vi "GUI_CH1_RXXXX_TCPIP.vi"() -> ()   [LabVIEW 2018]
uses:
  <resource>/objmgr/ni.dex.rc
panel:
  in  "stop 2":bool
  out "error out 3":errorcluster
  out "error out 2":errorcluster
  out "error out":errorcluster
  in  "stop":bool
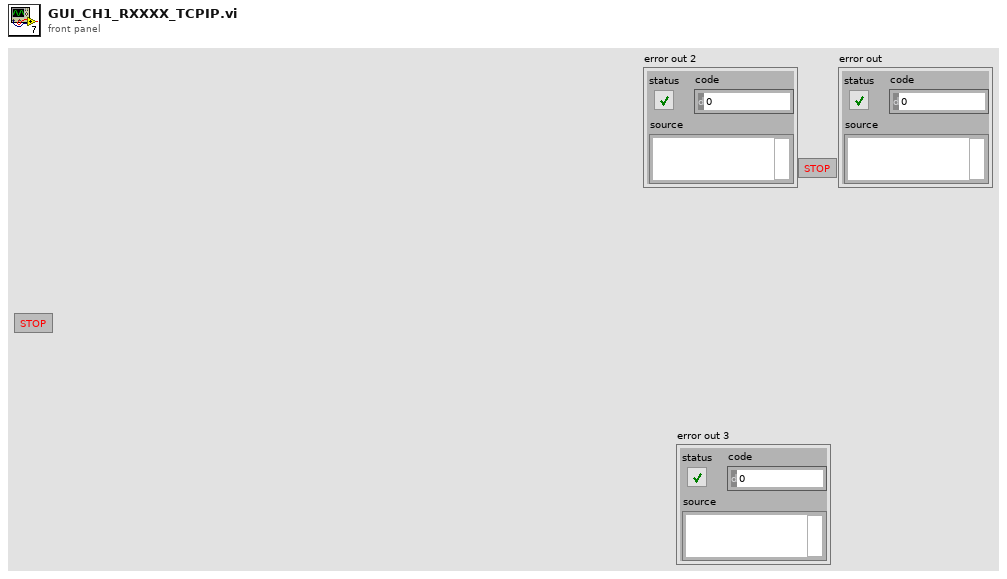
[diagram p1: front panel]
types:
  T1 = enum16{"Standard", "Buffered", "CRLF", "Immediate"}
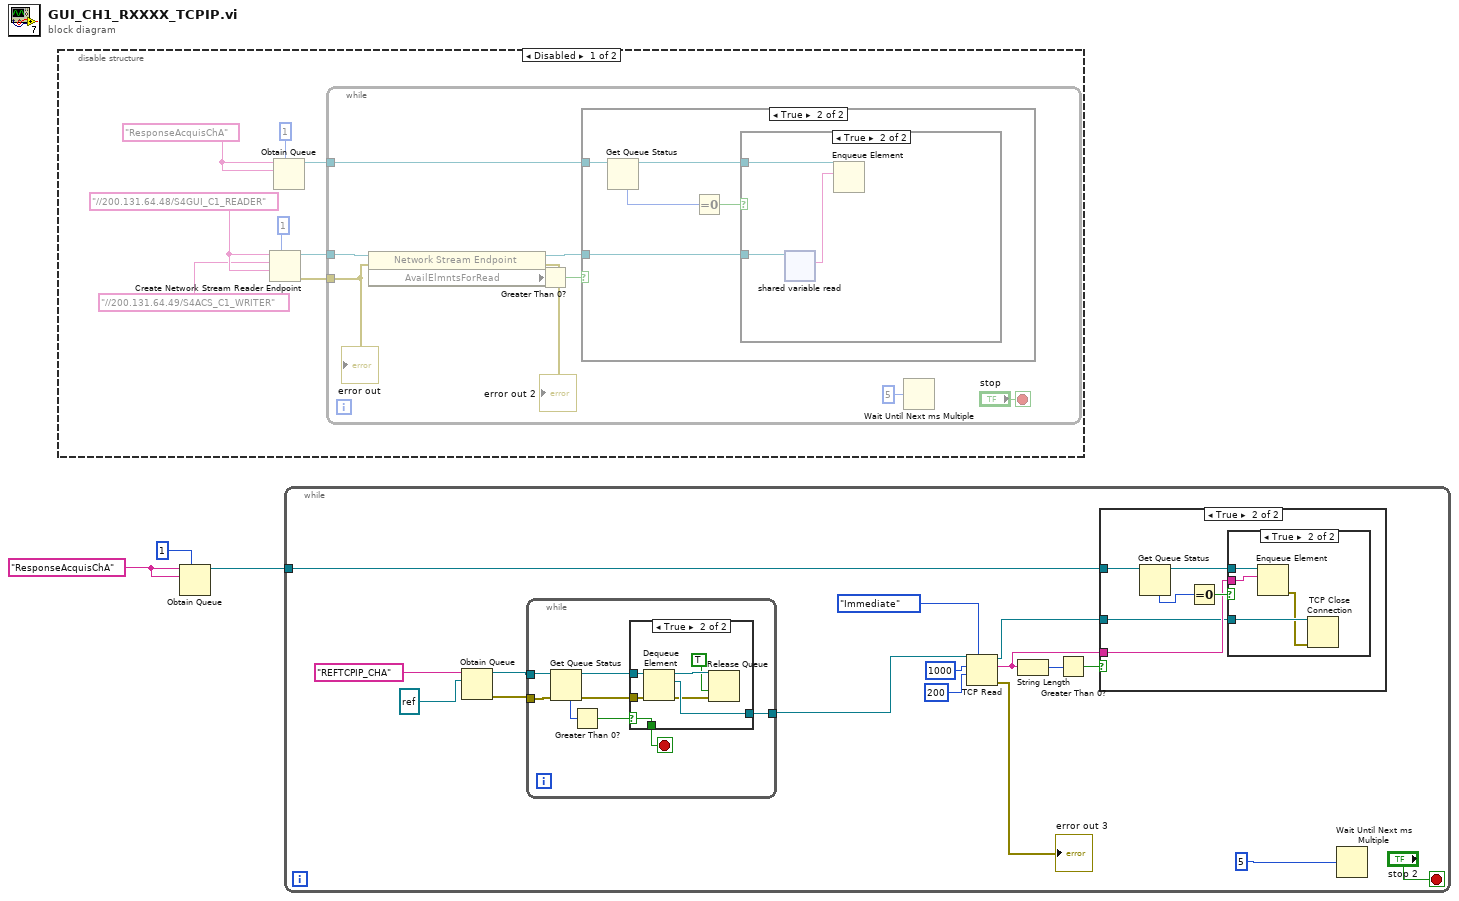
[diagram p0: block diagram]
diagram:
  w1 = "ResponseAcquisChA"
  n1 = disable-structure shown="Disabled" {
    frame Disabled {
      w6 = "//200.131.64.48/S4GUI_C1_READER"
      w11 = "ResponseAcquisChA"
      n2 = Create Network Stream Reader Endpoint(7:1 ("reader buffer size"), 9:w6, 10:"//200.131.64.49/S4ACS_C1_WRITER", 11:w6) -> (0:w5:errorcluster, 3:w8:refnum<k21>)  [unwired: 3 in]
      n3 = Obtain Queue(max queue size (-1, unlimited)=1, name (unnamed)=w11, element data type=w11) -> (queue out=w10:refnum<queue>)  [unwired: 2 in, 2 out]
      n4 = while {
        tunnel: w10 -> [w19]
        tunnel: w8 -> [w18]
        tunnel: w5 -> [w12]
        stop <- "stop" stop-if-true
        n5 = property class="Network Stream Endpoint"(reference=w18, error in=w12) -> (reference out=w17:refnum<k21>, error out=→"error out 2":errorcluster, "AvailElmntsForRead"=w16:i32)
        n6 = Greater Than 0?(x=w16) -> (x > 0?=w15:bool)
        n7 = case shown="True" w15 {
          tunnel: w19 -> [_ w22]
          tunnel: w17 -> [_ w25]
          frame False {
          }
          frame True {
            n8 = Get Queue Status(queue=w22) -> (queue out=w21:refnum<queue>, # elements in queue=w24:i32)  [unwired: 2 in, 6 out]
            n9 = Equal To 0?(x=w24) -> (x = 0?=w23:bool)
            n10 = case shown="True" w23 {
              tunnel: w25 -> [_ w28]
              tunnel: w21 -> [_ w26]
              frame False {
              }
              frame True {
                n11 = shared-variable-read(w28) -> (w27:string)  [unwired: 2 in, 3 out]
                n12 = Enqueue Element(queue=w26, element=w27) -> ()  [unwired: 2 in, 3 out]
              }
            }
          }
        }
        n13 = Wait Until Next ms Multiple(millisecond multiple=u32 5) -> ()  [unwired: 1 out]
        "error out" <- w12
      }
    }
    frame Enabled {
    }
  }
  n14 = Obtain Queue(max queue size (-1, unlimited)=1, name (unnamed)=w1, element data type=w1) -> (queue out=w3:refnum<queue>)  [unwired: 2 in, 2 out]
  n15 = while {
    tunnel: w3 -> [w43]
    stop <- "stop 2" stop-if-true
    n16 = Obtain Queue(name (unnamed)="REFTCPIP_CHA", element data type=refnum<k5> refnum ("connection ID out")) -> (queue out=w30:refnum<queue>, error out=w29:errorcluster)  [unwired: 3 in, 1 out]
    n17 = while {
      tunnel: [w47] -> w33
      tunnel: w30 -> [w46]
      tunnel: w29 -> [w45]
      stop <- w48 stop-if-true
      n18 = Get Queue Status(queue=w46, error in (no error)=w45) -> (queue out=w52:refnum<queue>, error out=w51:errorcluster, # elements in queue=w49:i32)  [unwired: 1 in, 5 out]
      n19 = Greater Than 0?(x=w49) -> (x > 0?=w50:bool)
      n20 = case shown="True" w50 {
        selector: w50 -> [w53 w58]
        tunnel: w52 -> [_ w60]
        tunnel: w51 -> [_ w59]
        tunnel: [w53 w58] -> w48
        tunnel: [_ w57] -> w47
        frame False {
        }
        frame True {
          n21 = Dequeue Element(queue=w60, error in (no error)=w59) -> (queue out=w56:refnum<queue>, element=w57:refnum<k5>, error out=w55:errorcluster)  [unwired: 1 in, 1 out]
          n22 = Release Queue(queue=w56, force destroy? (F)=TRUE, error in (no error)=w55) -> ()  [unwired: 3 out]
        }
      }
    }
    n23 = TCP Read(connection ID=w33, bytes to read=1000, 7:T1."Immediate" ("mode (standard)"), 9:200 ("bytes to read")) -> (connection ID out=w34:refnum<k5>, data out=w39:string, error out=→"error out 3":errorcluster)  [unwired: 1 in]
    n24 = String Length(string=w39) -> (length=w41:i32)
    n25 = Greater Than 0?(x=w41) -> (x > 0?=w40:bool)
    n26 = case shown="True" w40 {
      tunnel: w43 -> [_ w64]
      tunnel: w39 -> [_ w62]
      tunnel: w34 -> [_ w61]
      frame False {
      }
      frame True {
        n27 = Get Queue Status(queue=w64) -> (queue out=w63:refnum<queue>, # elements in queue=w66:i32)  [unwired: 2 in, 6 out]
        n28 = Equal To 0?(x=w66) -> (x = 0?=w65:bool)
        n29 = case shown="True" w65 {
          tunnel: w63 -> [_ w70]
          tunnel: w62 -> [_ w69]
          tunnel: w61 -> [_ w68]
          frame False {
          }
          frame True {
            n30 = Enqueue Element(queue=w70, element=w69) -> (error out=w67:errorcluster)  [unwired: 2 in, 2 out]
            n31 = TCP Close Connection(connection ID=w68, error in (no error)=w67) -> ()  [unwired: 1 in, 2 out]
          }
        }
      }
    }
    n32 = Wait Until Next ms Multiple(millisecond multiple=u32 5) -> ()  [unwired: 1 out]
  }
